vi "Set Cell.vi"(7 "Cell":refnum<class "Cell.lvclass">, 8 "error in":errorcluster, 9 "Column":i32, 10 "Row":i32, 11 "Sourcegrid in":refnum<class "SourceGrid.lvclass">) -> (0 "error out":errorcluster, 3 "Sourcegrid out":refnum<class "SourceGrid.lvclass">)   [LabVIEW 2024, in "SourceGrid.lvlib" / "SourceGrid.lvclass"]
doc: "Set the specified cell int he specified position."
uses:
  SourceGrid.lvclass
  Cells/Cell/Cell.lvclass
  SourceGrid.lvclass/SourceGrid.ctl
  Cells/Cell/Cell.lvclass/Cell.ctl
  D:/git/Sourcegrid-LabVIEW/dll/SourceGrid.dll
  dll/SourceGrid.dll
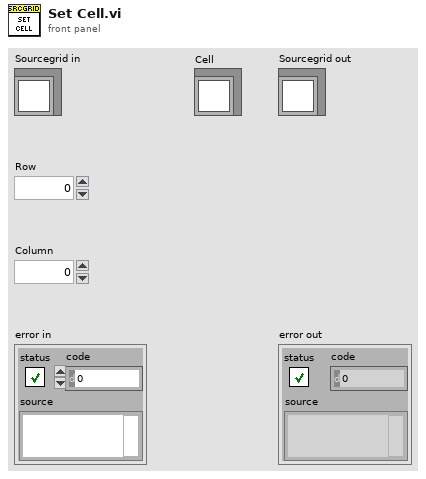
[diagram p1: front panel]
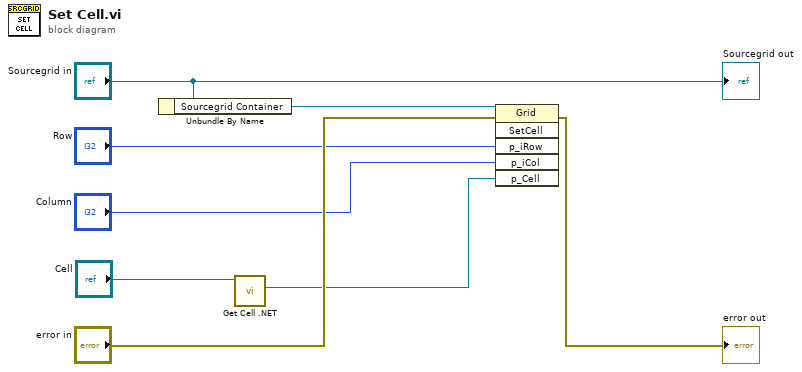
[diagram p0: block diagram]
diagram:
  n1 = Unbundle By Name("Sourcegrid in") -> ("Sourcegrid Container"=w8:refnum<k24>)
  n2 = call "Get Cell .NET.vi"("Cell in"="Cell") -> ("Cell .NET"=w4:refnum<k24>)  [unwired: 9 in, 1 out]
  n3 = invoke class="Grid" method="SetCell"(reference=w8, error in="error in", "p_iRow"="Row", "p_iCol"="Column", "p_Cell"=w4) -> (error out=→"error out":errorcluster)  [unwired: 1 in, 5 out]
  "Sourcegrid out" <- "Sourcegrid in"
